vi "256-bit CHDR Packetizer (Simple).vi"(6 "ready for output":bool, 7 "reset":bool, 8 "aurora frame length":u16, 9 "input valid":bool, 10 "header parameters":T1, 11 "data":bool[](array[boolean])) -> (0 "tlast":bool, 1 "output valid":bool, 2 "tkeep":bool[](array[boolean]), 3 "data out":bool[](array[boolean]), 4 "ready for input":bool)   [LabVIEW 2023, in "CHDR Support.lvlib"]
doc: "Inserts CHDR packet headers based on the provided aurora frame length. <b>Ready for Input</b> returns false if next data is a header."
uses:
  CHDR Support.lvlib
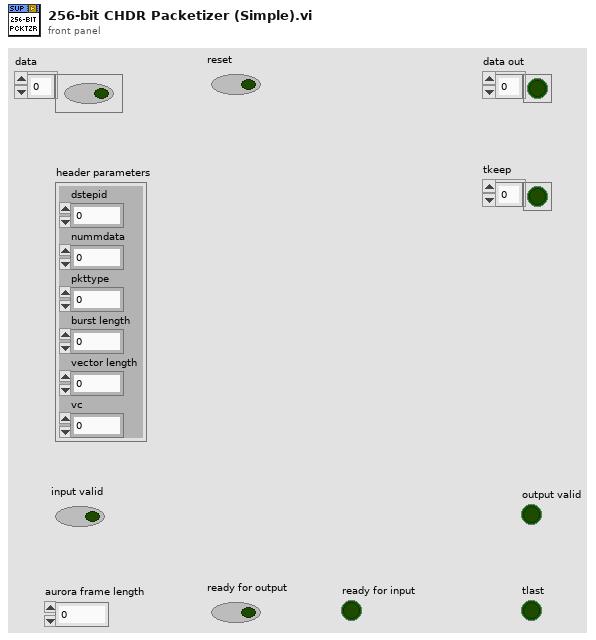
[diagram p1: front panel]
types:
  T1 = cluster{"dstepid":u16, "nummdata":fxp<+,5,5>, "pkttype":fxp<+,3,3>, "burst length":u16, "vector length":u16, "vc":fxp<+,6,6>}
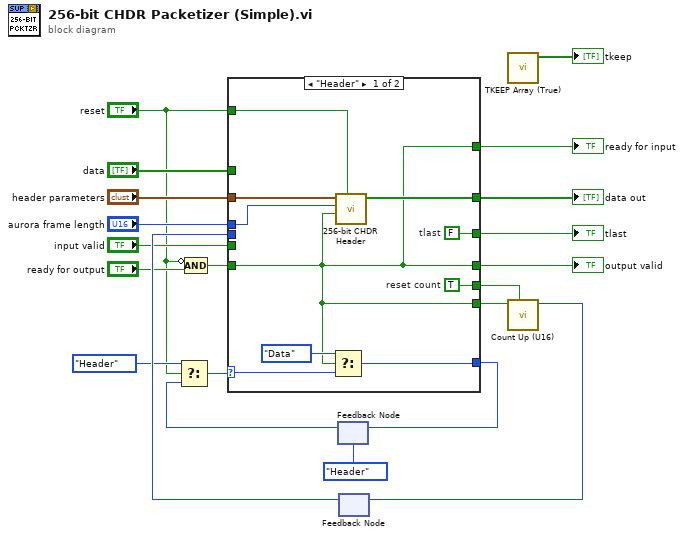
[diagram p0: block diagram]
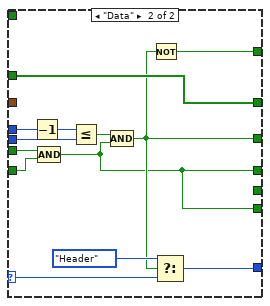
[diagram p2: hidden frame]
diagram:
  n1 = Compound Arithmetic op=AND(invert "reset", "ready for output") -> (w1:bool)
  n2 = feedback #1(enum16{"Header", "Data"}."Header") -> (w4:enum16{"Header", "Data"})
  n3 = Select(t=enum16{"Header", "Data"}."Header", s="reset", f=w4) -> (s? t:f=w5:enum16{"Header", "Data"})
  n4 = feedback #2() -> (w11:u16)  [unwired: 1 in]
  n5 = case shown="\"Header\"" w5 {
    selector: w5 -> [w27 w43]
    tunnel: [w22 w35] -> w21
    tunnel: "header parameters" -> [w31 _]
    tunnel: "reset" -> [w30 _]
    tunnel: w1 -> [w22 w37]
    tunnel: [w28 w44] -> w18
    tunnel: [w26 w41] -> w17
    tunnel: "aurora frame length" -> [w25 w40]
    tunnel: [w24 w34] -> w13
    tunnel: [w22 w33] -> w15
    tunnel: [w23 _] -> w7
    tunnel: [w22 w33] -> w8
    tunnel: "data" -> [_ w41]
    tunnel: w11 -> [_ w39]
    tunnel: "input valid" -> [_ w38]
    frame "Header" {
      w24 = FALSE  # tlast
      w23 = TRUE  # reset count
      n6 = Select(t=enum16{"Header", "Data"}."Data", s=w22, f=w27) -> (s? t:f=w28:enum16{"Header", "Data"})
      n7 = call "256-bit CHDR Header.vi"("reset"=w30, "ready for output"=w22, "aurora frame length"=w25, "header parameters"=w31) -> ("chdr header"=w26:bool[])  [unwired: 7 in]
    }
    frame "Data" {
      n8 = Decrement(x=w40) -> (x-1=w32:u16)
      n9 = Compound Arithmetic op=AND(w38, w37) -> (w33:bool)
      n10 = Less Or Equal?(x=w32, y=w39) -> (x <= y?=w36:bool)
      n11 = Compound Arithmetic op=AND(w36, w33) -> (w34:bool)
      n12 = Not(x=w34) -> (.not. x?=w35:bool)
      n13 = Select(t=enum16{"Header", "Data"}."Header", s=w34, f=w43) -> (s? t:f=w44:enum16{"Header", "Data"})
    }
  }
  "ready for input" <- w21
  "data out" <- w17
  "tlast" <- w13
  "output valid" <- w15
  n14 = feedback-in #1(w18) -> ()
  n15 = call "TKEEP Array (True).vi"() -> ("tkeep"=→"tkeep":bool[])  [unwired: 11 in]
  n16 = call "Count Up (U16).vi"("reset"=w7, "increment"=w8) -> ("count out"=w14:u16)  [unwired: 9 in]
  n17 = feedback-in #2(w14) -> ()
